vi "Curtin1_Search.vi"(9 "Old Files":T3[](array[typedef])) -> (1 "New Files":T3[](array[typedef]), 3 "Ok?":bool)   [LabVIEW 2022 SP3]
uses:
  <vilib>/Utility/miscctls.llb/LVSelectionTypeDef.ctl
  Mic/Mic_Global.vi
  Curtin1_Label.ctl
panel:
  out "cover":bool
  in  "Listing Order":T1(ring)
  in  "Tags":T2={"Pattern (eg. H,V)"="H,V", "File type"={"AvR"=TRUE, "AvC"=FALSE, "trf"=FALSE, "wav"=FALSE, "All"=FALSE}, "keywords 1"="", "keywords 2"="", "keywords 3"=""}
  out "# Files":i32
  out "AllFiles":path[](array[path])
  in  "Options":i32[](listbox)
  out "Files":path[](array[path])
  in  "Dialog":bool
  out "Subfolder":string
  in  "Search":bool
  out "Folder":cluster{"Folder Path":path, "tags":string[]}[](array[cluster])
  out "List":string
  in  "Cancel Button":bool
  in  "OK Button":bool
  # "Or"
  # "Or"
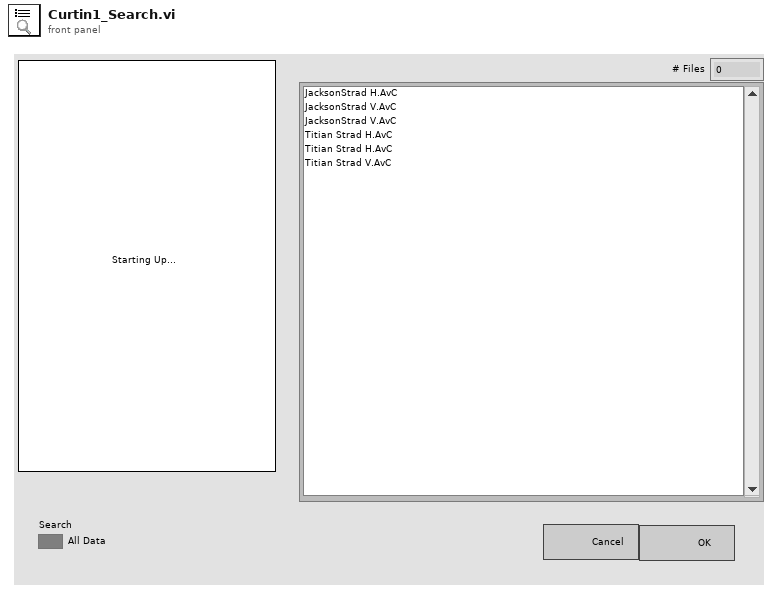
[diagram p1: front panel]
types:
  T1 = enum16{"Alphabetical", "Chronological", "Hit Strength (min to max)", "Hit Strength (max to min)"}
  T2 = cluster{"Pattern (eg. H,V)":string, "File type":cluster{"AvR":bool, "AvC":bool, "trf":bool, "wav":bool, "All":bool}, "keywords 1":string, "keywords 2":string, "keywords 3":string}
  T3 = typedef "Curtin1_Label.ctl" = cluster{"Show?":bool, "Name":string, "Color":u32, "Path":path, "Show Notes":bool, "correlate":bool}
  T4 = enum8{"Enabled", "Disabled", "Disabled and Grayed Out"}
  T5 = typedef "LVSelectionTypeDef.ctl" = cluster{"Selection Start":u32, "Selection End":u32}
  T6 = cluster{"Pattern (eg. H,V)":string, "File type":cluster{"AvR":bool, "AvC":bool, "trf":bool, "wfm":bool, "All":bool}, "keywords 1":string, "keywords 2":string, "keywords 3":string}
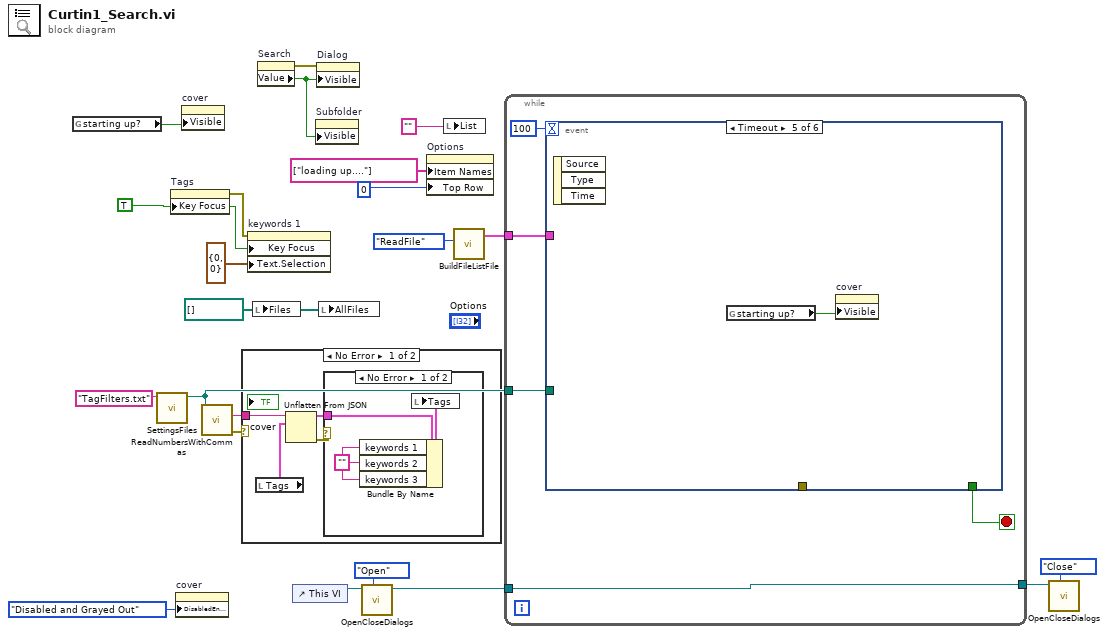
[diagram p0: block diagram]
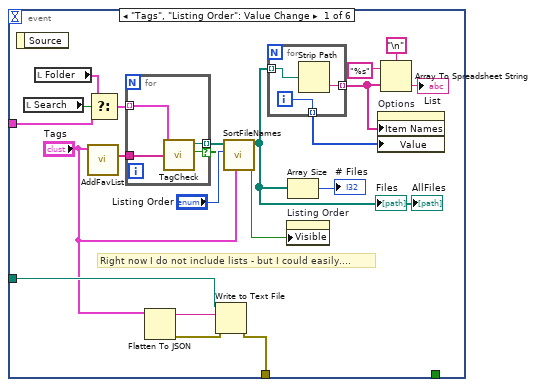
[diagram p4: hidden frame]
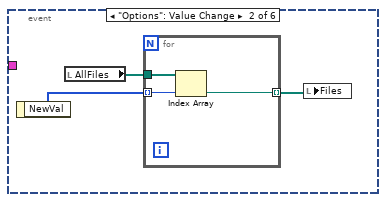
[diagram p5: hidden frame]
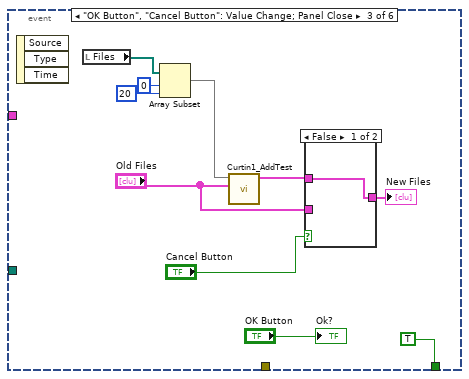
[diagram p6: hidden frame]
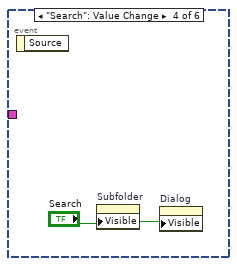
[diagram p8: hidden frame]
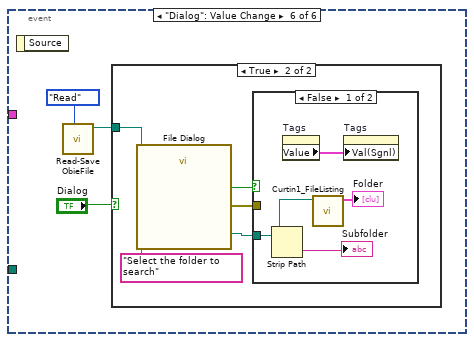
[diagram p9: hidden frame]
diagram:
  w5 = path[] [] ("Files")
  w14 = TRUE ("Visible")
  n1 = global read "Mic_Global.vi" "starting up?"() -> (w2:bool)
  n2 = call "SettingsFiles.vi"("settings file name"="TagFilters.txt" ("name or relative path")) -> ("file path"=w3:path)  [unwired: 9 in, 1 out]
  n3 = property on="Tags" class="Clust (strict)"("Key Focus"=w14) -> (error out=w13:errorcluster)  [unwired: 2 in, 1 out]
  n4 = property on="cover" class="Bool (strict)"("DisabledEnum"=T4."Disabled and Grayed Out" ("Disabled")) -> ()  [unwired: 2 in, 2 out]
  n5 = property on="cover" class="Bool (strict)"("Visible"=w2) -> ()  [unwired: 2 in, 2 out]
  n6 = call "ReadNumbersWithCommas.vi"("file (use dialog)"=w3) -> ("error out"=w11:errorcluster, "text"=w12:string)  [unwired: 7 in, 2 out]
  n7 = case shown="No Error" w11 {
    tunnel: w12 -> [w25 _]
    frame No Error {
      n8 = local read "Tags"() -> (w26:T2)
      n9 = Unflatten From JSON(JSON string=w25, type and defaults=w26) -> (value=w23:T2, error out=w24:errorcluster)  [unwired: 5 in]
      n10 = case shown="No Error" w24 {
        tunnel: w23 -> [w29 _]
        frame No Error {
          w28 = "" ("Tags 1")
          n11 = Bundle By Name(cluster=w29, "keywords 1"=w28, "keywords 2"=w28, "keywords 3"=w28) -> (w27:T2)
          n12 = local write "Tags"(w27) -> ()
        }
        frame Error {
        }
      }
    }
    frame Error {
    }
  }
  n13 = property on="keywords 1" class="Str"(error in=w13, "Key Focus"=w14, "Text.Selection"=T5 {"Selection Start"=0, "Selection End"=0}) -> ()  [unwired: 1 in, 2 out]
  n14 = local write "Files"(w5) -> ()
  n15 = property on="Search" class="Bool (strict)"() -> (error out=w18:errorcluster, "Value"=w17:bool)  [unwired: 2 in, 1 out]
  n16 = control-ref of="This VI"() -> (w9:refnum<vi>)
  n17 = property on="Subfolder" class="Str"("Visible"=w17) -> ()  [unwired: 2 in, 2 out]
  n18 = property on="Dialog" class="Bool"(error in=w18, "Visible"=w17) -> ()  [unwired: 1 in, 2 out]
  n19 = local write "AllFiles"(w5) -> ()
  n20 = call "OpenCloseDialogs.vi"("Task"=enum16{"Open", "Close"}."Open", "VI in"=w9) -> ("VI out"=w6:refnum<vi>)  [unwired: 8 in, 1 out]
  n21 = property on="Options" class="LstBox (strict)"("Item Names"=string[] ["loading up...."], "Top Row"=0) -> ()  [unwired: 2 in, 2 out]
  n22 = local write "List"("" ("List")) -> ()
  n23 = call "BuildFileListFile.vi"("Task"=enum16{"BuildFile", "ReadFile"}."ReadFile") -> ("Instruments"=w19:cluster{"Folder Path":path, "tags":string[]}[])  [unwired: 9 in, 1 out]
  n24 = while {
    tunnel: w19 -> [w33]
    tunnel: w3 -> [w32]
    tunnel: [w31] -> w7
    tunnel: w6 -> [w31]
    stop <- w34 stop-if-true
    n25 = event shown="[4] Timeout" {
      selector: _ -> [_ _ _ _ _ _]
      dyn-events: _ -> [_ _ _ _ _ _]
      timeout: 100 -> [_ _ _ _ _ _]
      tunnel: [_ _ TRUE _ _ _] -> w34
      tunnel: w33 -> [w42 _ _ _ _ _]
      tunnel: w32 -> [w48 _ _ _ _ _]
      tunnel: [w46 _ _ _ _ _] -> _
      event "Tags", "Listing Order": Value Change {
        # "Right now I do not include lists - but I could easily...."
        n26 = event-data() -> ()  [unwired: 1 in, 1 out]
        n27 = local read "Search"() -> (w43:bool)
        n28 = local read "Folder"() -> (w41:cluster{"Folder Path":path, "tags":string[]}[])
        n29 = call "AddFavList.vi"("Tags"="Tags") -> ("Tags"=w53:string[])  [unwired: 8 in, 2 out]
        n30 = Select(t=w41, s=w43, f=w42) -> (s? t:f=w40:cluster{"Folder Path":path, "tags":string[]}[])
        n31 = for {
          tunnel: w53 -> [w59]
          tunnel: [w61] -> w39 mode=indexing if=w60
          tunnel: w40 -> [w58] mode=indexing
          n32 = call "TagCheck.vi"("Tags"=w59, 11:w58) -> ("Good?"=w60:bool, "Path out"=w61:path)  [unwired: 8 in]
        }
        n33 = Flatten To JSON(anything="Tags") -> (JSON string=w49:string, 11:w47:errorcluster)  [unwired: 2 in]
        n34 = Write to Text File(file (use dialog)=w48, text=w49, error in=w47) -> (error out=w46:errorcluster)  [unwired: 1 in, 2 out]
        n35 = call "SortFileNames.vi"("Tags"="Tags", "Listing Order"="Listing Order", "Files in"=w39) -> ("wfm only?"=w35:bool, "Files out"=w38:path[])  [unwired: 7 in]
        "Files" <- w38
        "AllFiles" <- w38
        n36 = for {
          tunnel: w38 -> [w57] mode=indexing
          tunnel: [w56] -> w45 mode=indexing
          tunnel: [w55] -> w44 mode=indexing
          i -> [w55]
          n37 = Strip Path(path=w57) -> (name=w56:string)  [unwired: 1 out]
        }
        n38 = property on="Listing Order" class="Enum (strict)"("Visible"=w35) -> ()  [unwired: 2 in, 2 out]
        n39 = Array Size(array=w38) -> (size(s)=→"# Files":i32)
        n40 = property on="Options" class="LstBox (strict)"("Item Names"=w45, "Value"=w44) -> ()  [unwired: 2 in, 2 out]
        n41 = Array To Spreadsheet String(delimiter (Tab)="\n", array=w45, 3:"%s" ("format string")) -> (spreadsheet string=→"List":string)
      }
      event "Options": Value Change {
        n42 = event-data() -> ("NewVal"=w63:i32[])  [unwired: 1 in]
        n43 = local read "AllFiles"() -> (w64:path[])
        n44 = for {
          tunnel: w64 -> [w67]
          tunnel: w63 -> [w66] mode=indexing
          tunnel: [w65] -> w62 mode=indexing
          n45 = Index Array(array=w67, index=w66) -> (element=w65:path)
        }
        n46 = local write "Files"(w62) -> ()
      }
      event "OK Button", "Cancel Button": Value Change; Panel Close {
        n47 = event-data() -> ()  [unwired: 1 in, 3 out]
        n48 = local read "Files"() -> (w71:path[])
        n49 = Array Subset(array=w71, index=0, length=20) -> (w68:path[])
        n50 = call "Curtin1_AddTest.vi"("Old Files"="Old Files", "Selected Paths"=w68) -> ("New Files"=w75:T3[])  [unwired: 9 in]
        n51 = case shown="False" "Cancel Button" {
          tunnel: "Old Files" -> [_ w79]
          tunnel: w75 -> [w78 _]
          tunnel: [w78 w79] -> w74
          frame False {
          }
          frame True {
          }
        }
        "New Files" <- w74
        "Ok?" <- "OK Button"
      }
      event "Search": Value Change {
        n52 = event-data() -> ()  [unwired: 1 in, 1 out]
        n53 = property on="Subfolder" class="Str"("Visible"="Search") -> ()  [unwired: 2 in, 2 out]
        n54 = property on="Dialog" class="Bool"("Visible"="Search") -> ()  [unwired: 2 in, 2 out]
      }
      event Timeout {
        n55 = event-data() -> ()  [unwired: 1 in, 3 out]
        n56 = global read "Mic_Global.vi" "starting up?"() -> (w81:bool)
        n57 = property on="cover" class="Bool (strict)"("Visible"=w81) -> ()  [unwired: 2 in, 2 out]
      }
      event "Dialog": Value Change {
        n58 = event-data() -> ()  [unwired: 1 in, 1 out]
        n59 = call "Read-Save ObieFile.vi"("Task"=enum16{"Save", "Read"}."Read") -> ("DataPath Out"=w82:path)  [unwired: 8 in, 2 out]
        n60 = case shown="True" "Dialog" {
          tunnel: w82 -> [_ w86]
          frame False {
          }
          frame True {
            n61 = call "File Dialog"("start path"=w86, "prompt"="Select the folder to search" ("List")) -> ("selected path"=w89:path, "cancelled"=w88:bool, "error out"=w87:errorcluster)  [unwired: 10 in, 1 out]
            n62 = case shown="False" w88 {
              tunnel: w89 -> [w92 _]
              tunnel: w87 -> [_ _]
              frame False {
                n63 = Strip Path(path=w92) -> (name=→"Subfolder":string)  [unwired: 1 out]
                n64 = property on="Tags" class="Clust (strict)"() -> ("Value"=w90:T6)  [unwired: 2 in, 2 out]
                n65 = call "Curtin1_FileListing.vi"("Folder Path"=w92) -> ("Array"=→"Folder":cluster{"Folder Path":path, "tags":string[]}[])  [unwired: 10 in]
                n66 = property on="Tags" class="Clust (strict)"("Val(Sgnl)"=w90) -> ()  [unwired: 2 in, 2 out]
              }
              frame True {
              }
            }
          }
        }
      }
    }
  }
  n67 = call "OpenCloseDialogs.vi"("Task"=enum16{"Open", "Close"}."Close", "VI in"=w7) -> ()  [unwired: 8 in, 2 out]
